vi "Clear.vi"(0 "Display State In":T1={"logTable"=refnum, "max items"=500, "displaydata"=[], "data"=[], "Auto Scroll"=TRUE, "current item"=500, "col headers"=[], "Add to Top"=TRUE, "Auto resize"=TRUE, "col size"=[], "filters"=[], "color cells"=[]}, 9 "Container State":T3, 11 "error in (no error)":errorcluster) -> (4 "Display State Out":T1={"logTable"=refnum, "max items"=500, "displaydata"=[], "data"=[], "Auto Scroll"=TRUE, "current item"=500, "col headers"=[], "Add to Top"=TRUE, "Auto resize"=TRUE, "col size"=[], "filters"=[], "color cells"=[]}, 15 "error out":errorcluster)   [LabVIEW 2017, in "UI-DisplayTable(dev).xctl"]
uses:
  UI-DisplayTable(dev).xctl
  <vilib>/_xctls/Container State.ctl
  State.ctl
  Support/DEF-Filter.ctl
  <vilib>/_xctls/XControlSupport.lvlib
types:
  T1 = typedef "UI-DisplayTable(dev).xctl/State.ctl" = cluster{"logTable":refnum<vi>, "max items":i32, "displaydata":string[][], "data":string[][], "Auto Scroll":bool, "current item":i32, "col headers":string[], "Add to Top":bool, "Auto resize":bool, "col size":i32[], "filters":T2[], "color cells":cluster{"color cell":cluster{"Column":string, "Value":string, "Highlight Column":string}, "Color Box":u32}[]}
  T2 = typedef "UI-DisplayTable(dev).xctl/DEF-Filter.ctl" = cluster{"column":string, "value":string[]}
  T3 = typedef "XControlSupport.lvlib/Container State.ctl" = cluster{"Indicator?":bool, "Run Mode?":bool, " Refnum":refnum<vi>}
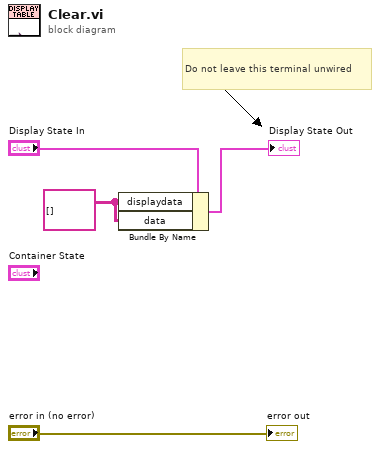
[diagram p0: block diagram]
diagram:
  w1 = string[][] [] ("displaydata")
  # "Do not leave this terminal unwired"
  n1 = Bundle By Name(cluster="Display State In", "displaydata"=w1, "data"=w1) -> (→"Display State Out":T1)
  "error out" <- "error in (no error)"
